vi "SwissSPAD Live_Upload Bitfile.vi"(8 "error in (no error)":errorcluster, 10 "FPGA bitfile Path":path, 11 "okCFrontPanel Device Refnum":refnum<k24>) -> (0 "error out":errorcluster, 3 "okCFrontPanel Device Refnum":refnum<k24>)   [LabVIEW 2021]
uses:
  D:/UCLA Thinkpad Google Drive/LabVIEW 2021 SP1/builds/SwissSPAD Live Distribution/Opal Kelly/C# Wrapper/v5.0.2/libFrontPanel-csharp.dll
  Opal Kelly/C# Wrapper/v5.0.2/libFrontPanel-csharp.dll
  Opal Kelly/C# Wrapper/okFrontPanelC#Wrapper.lvlib
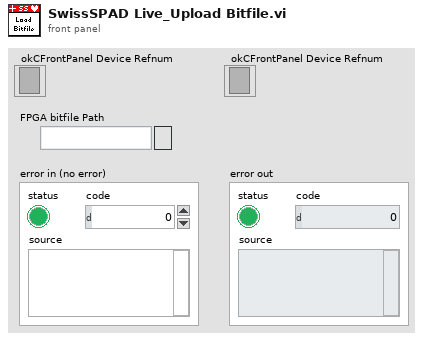
[diagram p1: front panel]
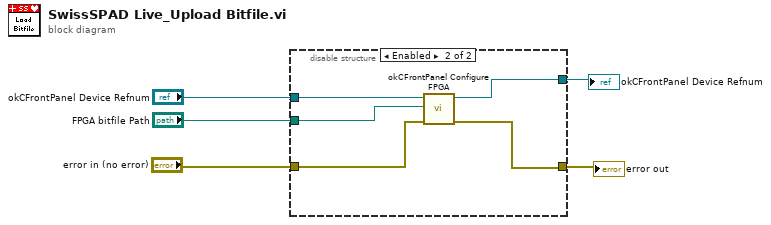
[diagram p0: block diagram]
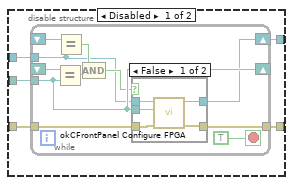
[diagram p2: hidden frame]
diagram:
  n1 = disable-structure shown="Enabled" {
    disable-tunnel: "FPGA bitfile Path" -> [w10 w32]
    disable-tunnel: "okCFrontPanel Device Refnum" -> [w9 w33]
    disable-tunnel: "error in (no error)" -> [w8 w29]
    disable-tunnel: [w7 w30] -> w2
    disable-tunnel: [w6 w31] -> w1
    frame Disabled {
      n2 = while {
        tunnel: w10 -> [w18]
        tunnel: w9 -> [w11]
        shift-right: [w12] -> w6
        shift-left: _ -> [w20]
        shift-right: [w18] -> _
        shift-left: _ -> [w19]
        tunnel: w8 -> [w17]
        tunnel: [w16] -> w7
        stop <- TRUE stop-if-true
        n3 = Equal?(x=w19, y=w18) -> (x = y?=w15:bool)
        n4 = Equal?(x=w20, y=w11) -> (x = y?=w14:bool)
        n5 = Compound Arithmetic op=AND(w14, w15) -> (w13:bool)
        n6 = case shown="False" w13 {
          tunnel: w18 -> [w26 _]
          tunnel: w17 -> [w25 w28]
          tunnel: [w24 w28] -> w16
          tunnel: w11 -> [w23 w27]
          tunnel: [w22 w27] -> w12
          frame False {
            n7 = call "okCFrontPanel Configure FPGA.vi"("error in (no error)"=w25, "FPGA bitfile Path"=w26, "okCFrontPanel Device Refnum"=w23) -> ("error out"=w24:errorcluster, "okCFrontPanel Device Refnum"=w22:refnum<k24>)  [unwired: 7 in]
          }
          frame True {
          }
        }
      }
    }
    frame Enabled {
      n8 = call "okCFrontPanel Configure FPGA.vi"("error in (no error)"=w29, "FPGA bitfile Path"=w32, "okCFrontPanel Device Refnum"=w33) -> ("error out"=w30:errorcluster, "okCFrontPanel Device Refnum"=w31:refnum<k24>)  [unwired: 7 in]
    }
  }
  "okCFrontPanel Device Refnum" <- w1
  "error out" <- w2
